vi "Print.vi"(8 "Error In":errorcluster, 11 "reference in":refnum<class "Client.lvclass">) -> (0 "Error Out":errorcluster, 3 "reference out":refnum<class "Client.lvclass">)   [LabVIEW 2020, in "Client.lvclass"]
uses:
  Client.lvclass
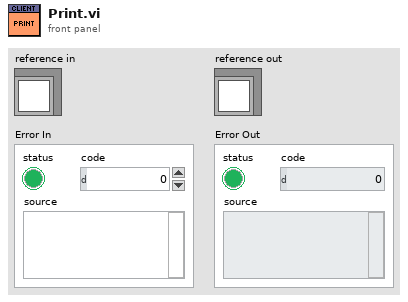
[diagram p1: front panel]
types:
  T1 = typedef "Client.lvclass/ObjectAttributes.ctl" = cluster{"_menus":refnum<class "MenuComponent.lvclass">}
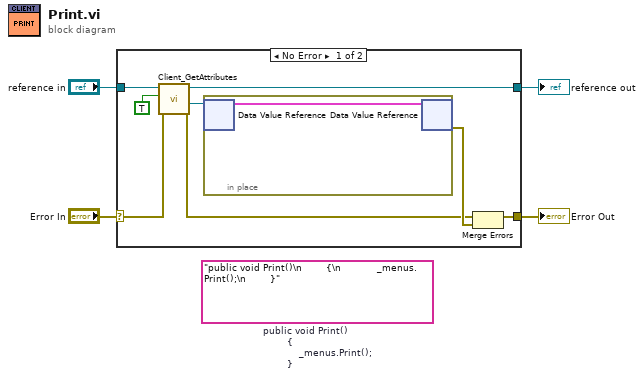
[diagram p0: block diagram]
diagram:
  (unwired) "public void Print()\n        {\n            _menus.Print();\n        }"  # public void Print()         {             _menus.Print();         }
  n1 = case shown="No Error" "Error In" {
    selector: "Error In" -> [w11 w15]
    tunnel: [w8 w15] -> w3
    tunnel: [w9 w14] -> w1
    tunnel: "reference in" -> [w12 w14]
    frame No Error {
      n2 = call "Client_GetAttributes.vi"("error in (no error)"=w11, "OnlyGetDvrReference(False)"=TRUE, "reference in"=w12) -> ("error out"=w6:errorcluster, "DataRef"=w7:refnum<data-value>, "reference out"=w9:refnum<class "Client.lvclass">)  [unwired: 5 in, 1 out]
      n3 = in-place {
        n4 = in-place-dvr #1(w7) -> (w13:T1)  [unwired: 1 out]
        n5 = in-place-dvr #1(w13) -> (w10:errorcluster)  [unwired: 1 out]
      }
      n6 = Merge Errors(w6, w10) -> (w8:errorcluster)
    }
    frame Error {
    }
  }
  "Error Out" <- w3
  "reference out" <- w1
